vi "kvCanTranslateBaud.vi"(0 "error in (no error)":errorcluster, 4 "Baud Rate":i32(ring) items=["Classic 1M", "Classic 500K", "Classic 250K", "Classic 125K", "Classic 100K", "Classic 62K", "Classic 50K", "Classic 83K", "FD 500K ", "FD 1M", "FD 2M", "FD 4M", "FD 8M"]) -> (1 "Sync Mode":u32, 2 "Number of Sampling Points":u32, 3 "error out":errorcluster, 5 "CAN Bus Frequency":u32, 6 "Time Segment 1":u32, 7 "Time Segment 2":u32, 8 "Synchronization Jump Width":u32)   [LabVIEW 2023]
doc: "This function translates the standard KVaser CAN BAUD_xxx constants to their corresponding bus parameter values."
uses:
  canlib32.dll
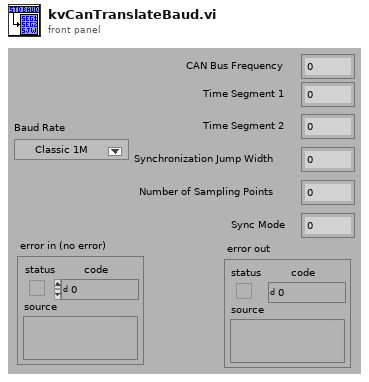
[diagram p1: front panel]
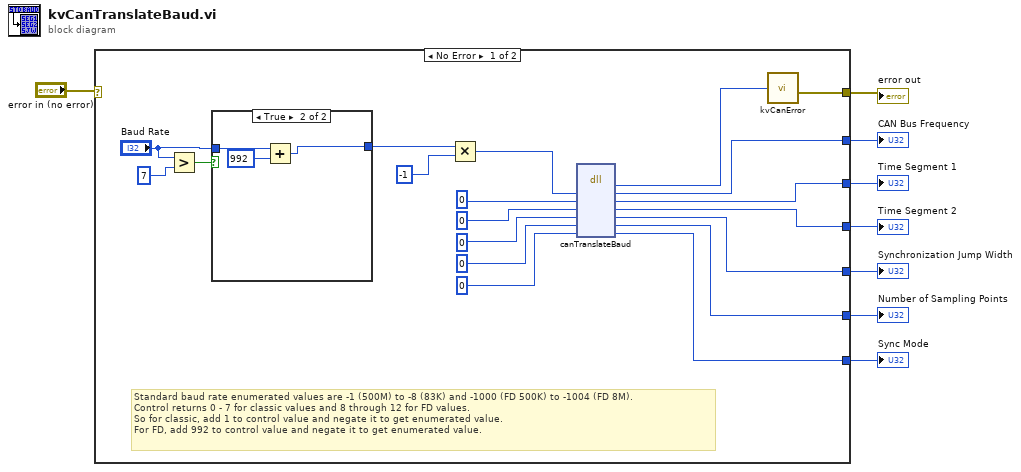
[diagram p0: block diagram]
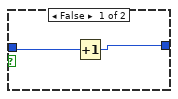
[diagram p2: hidden frame]
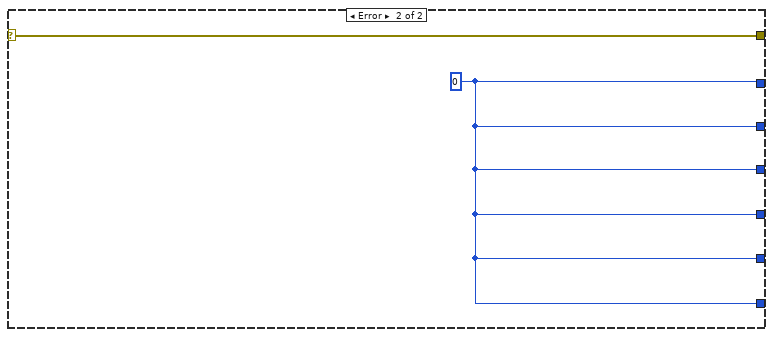
[diagram p3: hidden frame]
diagram:
  n1 = case shown="No Error" "error in (no error)" {
    selector: "error in (no error)" -> [_ w34]
    tunnel: [w19 w34] -> w7
    tunnel: [w18 w33] -> w6
    tunnel: [w17 w33] -> w5
    tunnel: [w16 w33] -> w4
    tunnel: [w15 w33] -> w3
    tunnel: [w14 w33] -> w2
    tunnel: [w13 w33] -> w1
    frame No Error {
      # "Standard baud rate enumerated values are -1 (500M) to -8 (83K) and -1000 (FD 500K) to -1004 (FD 8M).\nControl returns 0 - 7 for classic values and 8 through 12 for FD values.\nSo for classic, add 1 to control value and negate it to get enumerated value.\nFor FD, add 992 to control value and negate it to get enumerated value."
      n2 = Greater?(x="Baud Rate", y=7) -> (0:w11:bool)
      n3 = case shown="True" w11 {
        tunnel: "Baud Rate" -> [w29 w32]
        tunnel: [w28 w31] -> w9
        frame False {
          n4 = Increment(x=w29) -> (x+1=w28:i32)
        }
        frame True {
          n5 = Add(x=w32, y=992) -> (x+y=w31:i32)
        }
      }
      n6 = Multiply(x=w9, y=-1) -> (x*y=w22:i32)
      n7 = dll-call lib="canlib32.dll" fn="canTranslateBaud" label="Call Library Function"("freq"=w22, "tseg1"=0, "tseg2"=0, "sjw"=0, "nosamp"=0, "syncmode"=0) -> (w21:i32, "freq"=w18:i32, "tseg1"=w17:i32, "tseg2"=w16:i32, "sjw"=w15:i32, "nosamp"=w14:i32, "syncmode"=w13:i32)  [unwired: 3 in, 2 out]
      n8 = call "kvCanError.vi"("error code"=w21) -> ("error out"=w19:errorcluster)
    }
    frame Error {
      w33 = 0
    }
  }
  "Time Segment 1" <- w5
  "Time Segment 2" <- w4
  "Synchronization Jump Width" <- w3
  "Number of Sampling Points" <- w2
  "Sync Mode" <- w1
  "CAN Bus Frequency" <- w6
  "error out" <- w7
